vi "Carica sensori canale.vi"(7 "knob":refnum<vi>[](array[refnum]), 8 "error in (no error)":errorcluster, 9 "BANCO":i32, 10 "Array 2":refnum<vi>[](array[refnum]), 11 "Array":refnum<vi>[](array[refnum])) -> (0 "canale--sensore":string[][](array[string]), 1 "sens mand-asp-premist":T2(array[cluster]), 2 "Portate":T2(array[cluster]), 4 "SOMMA":bool)   [LabVIEW 2019]
uses:
  <vilib>/Utility/file.llb/Read Delimited Spreadsheet (string).vi
panel:
  in  "Unità di Misura":T1
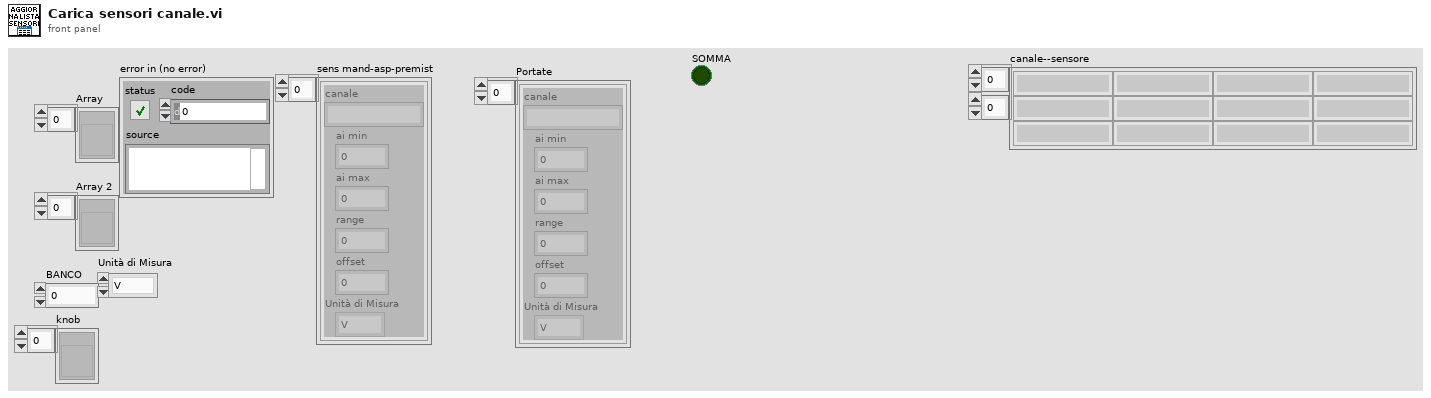
[diagram p1: front panel]
types:
  T1 = typedef "UnitàMisura.ctl" = enum16{"V", "mA", "Bar", "RPM", "m3/s", "m3/min", "m3/h", "l/s", "l/min", "in3/min", "ft3/min", "gpm", "igpm", "igph", "%", "°C", "m", "Nm", "A"}
  T2 = cluster{"canale":string, "ai min":dbl, "ai max":dbl, "range":dbl, "offset":dbl, "Unità di Misura":T1}[]
  T3 = cluster{"canale":string, "ai min":dbl, "ai max":dbl, "range":dbl, "offset":dbl, "Unità di Misura":T1}
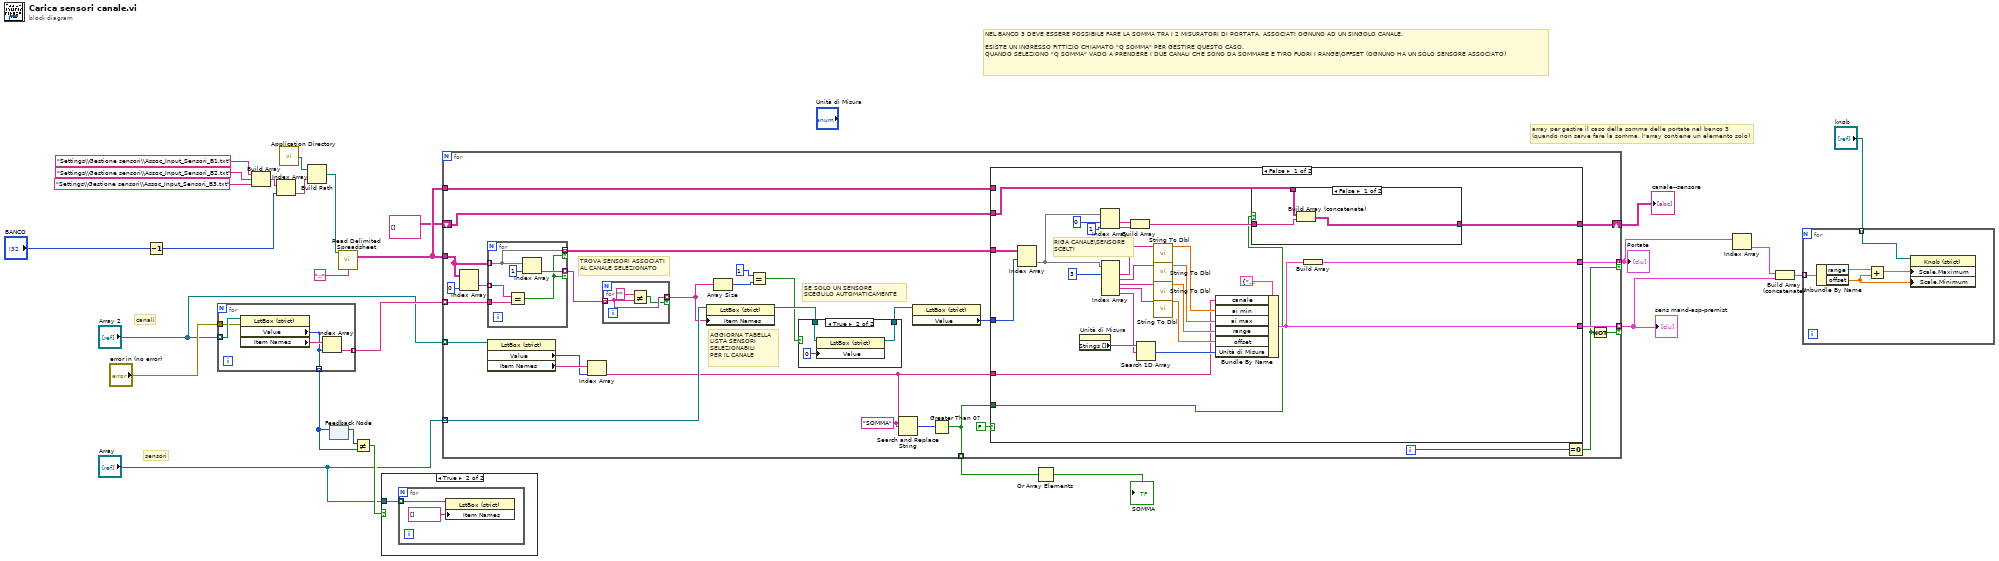
[diagram p0: block diagram]
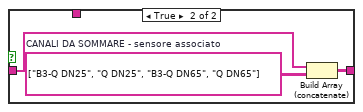
[diagram p3: hidden frame]
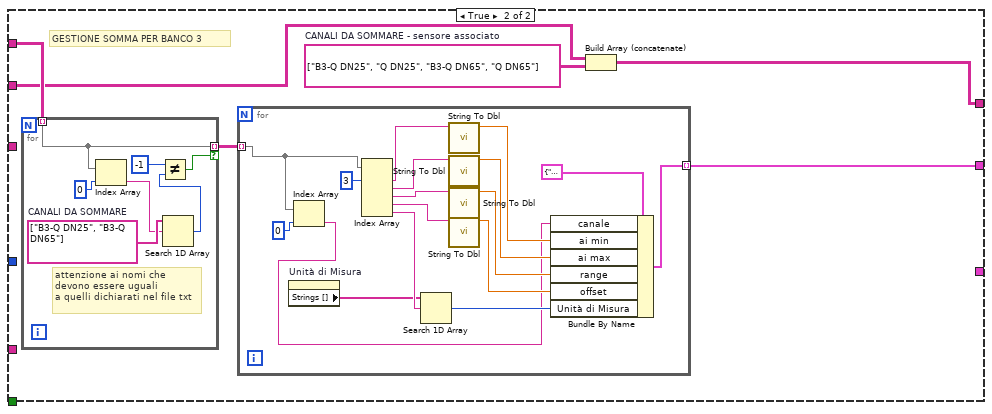
[diagram p4: hidden frame]
diagram:
  # "array per gestire il caso della somma delle portate nel banco 3\n(quando non serve fare la somma, l'array contiene un elemento solo)"
  # "NEL BANCO 3 DEVE ESSERE POSSIBILE FARE LA SOMMA TRA I 2 MISURATORI DI PORTATA, ASSOCIATI OGNUNO AD UN SINGOLO CANALE.\n\nESISTE UN INGRESSO FITTIZIO CHIAMATO \"Q SOMMA\" PER GESTIRE QUESTO CASO.\nQUANDO SELEZIONO \"Q SOMMA\" VADO A PRENDERE I DUE CANALI CHE SONO DA SOMMARE E TIRO FUORI I RANGE\\OFFSET (OGNUNO HA UN SOLO SENSORE ASSOCIATO)"
  # "sensori"
  # "canali"
  n1 = Decrement(x="BANCO") -> (x-1=w13:i32)
  n2 = for {
    tunnel: "Array 2" -> [w32] mode=indexing
    tunnel: [w30] -> w22 mode=indexing
    tunnel: [w29] -> w25 mode=indexing
    tunnel: "error in (no error)" -> [w28]
    n3 = property class="LstBox (strict)"(reference=w32, error in=w28) -> ("Value"=w29:i32, "Item Names"=w31:string[])  [unwired: 2 out]
    n4 = Index Array(array=w31, index=w29) -> (element=w30:string)
  }
  n5 = Build Array("Settings\\Gestione sensori\\Assoc_Input_Sensori_B1.txt" ("name or relative path"), "Settings\\Gestione sensori\\Assoc_Input_Sensori_B2.txt" ("name or relative path"), "Settings\\Gestione sensori\\Assoc_Input_Sensori_B3.txt" ("name or relative path")) -> (w20:string[])
  n6 = Index Array(array=w20, index=w13) -> (element=w16:string)
  n7 = call <vilib>:"Application Directory.vi"() -> ("Application Directory"=w17:path)
  n8 = Build Path(base path=w17, name or relative path=w16) -> (appended path=w15:path)
  n9 = feedback #1() -> (w24:i32[])  [unwired: 1 in]
  n10 = feedback-in #1(w25) -> ()
  n11 = call-poly <vilib>:"Read Delimited Spreadsheet.vi"("file path (dialog if empty)"=w15, "delimiter (\\t)"="::" ("delimiter (\\t)")) -> ("all rows"=w10:string[][])  [unwired: 8 in, 5 out]
  n12 = Not Equal?(x=w24, y=w25) -> (x != y?=w27:bool)
  n13 = case shown="True" w27 {
    tunnel: "Array" -> [_ w33]
    frame False {
    }
    frame True {
      n14 = for {
        tunnel: w33 -> [w35] mode=indexing
        n15 = property class="LstBox (strict)"(reference=w35, "Item Names"=string[] []) -> ()  [unwired: 1 in, 2 out]
      }
    }
  }
  n16 = for {
    tunnel: "Array" -> [w61] mode=indexing
    tunnel: w10 -> [w62]
    tunnel: w22 -> [w65] mode=indexing
    tunnel: [w60] -> w3 mode=indexing if=w41
    tunnel: "Array 2" -> [w50] mode=indexing
    tunnel: [w44] -> w5 mode=concatenating if=w42
    tunnel: w10 -> [w40]
    shift-right: [w39] -> w8
    shift-left: string[][] [] -> [w38]
    tunnel: [w36] -> w7 mode=indexing
    i -> [w43]
    w46 = "SOMMA" ("search string")
    # "SE SOLO UN SENSORE\nSCEGLILO AUTOMATICAMENTE"
    # "AGGIORNA TABELLA\nLISTA SENSORI\nSELEZIONABILI\nPER IL CANALE"
    # "TROVA SENSORI ASSOCIATI\nAL CANALE SELEZIONATO"
    n17 = Index Array(array=w62, index (col)=0 ("index")) -> (element=w63:string[])  [unwired: 1 in]
    n18 = for {
      tunnel: w65 -> [w141]
      tunnel: w63 -> [w140] mode=indexing
      tunnel: w62 -> [w137] mode=indexing
      tunnel: [w138] -> w52 mode=indexing if=w136
      tunnel: [w137] -> w59 mode=indexing if=w136
      n19 = Equal?(x=w140, y=w141) -> (x = y?=w136:bool)
      n20 = Index Array(array=w137, index=1) -> (element=w138:string)
    }
    n21 = property class="LstBox (strict)"(reference=w50) -> ("Value"=w48:i32, "Item Names"=w49:string[])  [unwired: 1 in, 2 out]
    n22 = Index Array(array=w49, index=w48) -> (element=w47:string)
    n23 = for {
      tunnel: w52 -> [w130] mode=indexing
      tunnel: [w130] -> w51 mode=indexing if=w129
      n24 = Not Equal?(x="", y=w130) -> (x != y?=w129:bool)
    }
    n25 = property class="LstBox (strict)"(reference=w61, "Item Names"=w51) -> (reference out=w57:refnum<vi>)  [unwired: 1 in, 1 out]
    n26 = Array Size(array=w51) -> (size(s)=w55:i32)
    n27 = Equal?(x=1, y=w55) -> (x = y?=w53:bool)
    n28 = case shown="True" w53 {
      tunnel: w57 -> [w132 w135]
      tunnel: [w132 w134] -> w56
      frame False {
      }
      frame True {
        n29 = property class="LstBox (strict)"(reference=w135, "Value"=0) -> (reference out=w134:refnum<vi>)  [unwired: 1 in, 1 out]
      }
    }
    n30 = Search and Replace String(input string=w47, search string=w46, replace string=w46) -> (number of replacements=w45:i32)  [unwired: 5 in, 3 out]
    n31 = property class="LstBox (strict)"(reference=w56) -> ("Value"=w58:i32)  [unwired: 1 in, 2 out]
    n32 = Greater Than 0?(x=w45) -> (x > 0?=w36:bool)
    n33 = case shown="False" FALSE {
      tunnel: [w76 _] -> w60
      tunnel: w59 -> [w91 _]
      tunnel: w58 -> [w90 _]
      tunnel: w47 -> [w77 _]
      tunnel: [w75 w99] -> w44
      tunnel: w40 -> [_ w103]
      tunnel: [w67 w101] -> w39
      tunnel: w38 -> [w69 w100]
      tunnel: w36 -> [w66 _]
      frame False {
        # "RIGA CANALE\\SENSORE\nSCELTI"
        n34 = Index Array(array=w91, index (row)=w90) -> (element=w74:string[])  [unwired: 1 in]
        n35 = property on="Unità di Misura" class="Enum (strict)"() -> ("Strings []"=w86:string[])  [unwired: 2 in, 2 out]
        n36 = Index Array(array=w74, index #1=0 ("index"), index #2=1 ("index")) -> (element #1=w70:string, element #2=w71:string)
        n37 = Index Array(array=w74, index #1=3 ("index")) -> (element #1=w88:string, element #2=w83:string, element #3=w81:string, element #4=w79:string, element #5=w85:string)  [unwired: 4 in]
        n38 = Build Array(w70, w71) -> (w68:string[])
        n39 = Search 1D Array(1D array=w86, element=w85) -> (index of element=w84:i32)  [unwired: 1 in]
        n40 = call "String To Dbl.vi"("String"=w88) -> ("Numeric"=w87:dbl)  [unwired: 10 in]
        n41 = call "String To Dbl.vi"("String"=w83) -> ("Numeric"=w82:dbl)  [unwired: 10 in]
        n42 = call "String To Dbl.vi"("String"=w81) -> ("Numeric"=w80:dbl)  [unwired: 10 in]
        n43 = call "String To Dbl.vi"("String"=w79) -> ("Numeric"=w78:dbl)  [unwired: 10 in]
        n44 = Bundle By Name(cluster=T3 {"canale"="", "ai min"=0.0, "ai max"=0.0, "range"=0.0, "offset"=0.0, "Unità di Misura"=enum."V"} ("portata"), "canale"=w77, "ai min"=w87, "ai max"=w82, "range"=w80, "offset"=w78, "Unità di Misura"=w84) -> (w76:T3)
        n45 = case shown="False" w66 {
          tunnel: w69 -> [w95 _]
          tunnel: w68 -> [w94 w97]
          tunnel: [w93 w96] -> w67
          frame False {
            n46 = Build Array (concatenate)(w95, w94) -> (w93:string[][])
          }
          frame True {
            w98 = string[][] [["B3-Q DN25", "Q DN25"], ["B3-Q DN65", "Q DN65"]]  # CANALI DA SOMMARE - sensore associato
            n47 = Build Array (concatenate)(w97, w98) -> (w96:string[][])
          }
        }
        n48 = Build Array(w76) -> (w75:T2)
      }
      frame True {
        w102 = string[][] [["B3-Q DN25", "Q DN25"], ["B3-Q DN65", "Q DN65"]]  # CANALI DA SOMMARE - sensore associato
        # "GESTIONE SOMMA PER BANCO 3"
        n49 = for {
          tunnel: [w105] -> w104 mode=indexing if=w108
          tunnel: w103 -> [w105] mode=indexing
          w110 = string[] ["B3-Q DN25", "B3-Q DN65"]  # CANALI DA SOMMARE
          # "attenzione ai nomi che \ndevono essere uguali\na quelli dichiarati nel file txt"
          n50 = Index Array(array=w105, index=0) -> (element=w109:string)
          n51 = Search 1D Array(1D array=w110, element=w109) -> (index of element=w107:i32)  [unwired: 1 in]
          n52 = Not Equal?(x=-1, y=w107) -> (x != y?=w108:bool)
        }
        n53 = for {
          tunnel: [w116] -> w99 mode=indexing
          tunnel: w104 -> [w114] mode=indexing
          n54 = property on="Unità di Misura" class="Enum (strict)"() -> ("Strings []"=w112:string[])  [unwired: 2 in, 2 out]
          n55 = Index Array(array=w114, index=0) -> (element=w113:string)
          n56 = Index Array(array=w114, index #1=3 ("index")) -> (element #1=w126:string, element #2=w122:string, element #3=w120:string, element #4=w118:string, element #5=w124:string)  [unwired: 4 in]
          n57 = Search 1D Array(1D array=w112, element=w124) -> (index of element=w123:i32)  [unwired: 1 in]
          n58 = call "String To Dbl.vi"("String"=w126) -> ("Numeric"=w125:dbl)  [unwired: 10 in]
          n59 = call "String To Dbl.vi"("String"=w122) -> ("Numeric"=w121:dbl)  [unwired: 10 in]
          n60 = call "String To Dbl.vi"("String"=w120) -> ("Numeric"=w119:dbl)  [unwired: 10 in]
          n61 = call "String To Dbl.vi"("String"=w118) -> ("Numeric"=w117:dbl)  [unwired: 10 in]
          n62 = Bundle By Name(cluster=T3 {"canale"="", "ai min"=0.0, "ai max"=0.0, "range"=0.0, "offset"=0.0, "Unità di Misura"=enum."V"} ("portata"), "canale"=w113, "ai min"=w125, "ai max"=w121, "range"=w119, "offset"=w117, "Unità di Misura"=w123) -> (w116:T3)
        }
        n63 = Build Array (concatenate)(w100, w102) -> (w101:string[][])
      }
    }
    n64 = Equal To 0?(x=w43) -> (x = 0?=w42:bool)
    n65 = Not(x=w42) -> (.not. x?=w41:bool)
  }
  "sens mand-asp-premist" <- w3
  "Portate" <- w5
  "canale--sensore" <- w8
  n66 = Or Array Elements(Boolean array=w7) -> (logical OR=→"SOMMA":bool)
  n67 = Index Array(array=w5) -> (element=w4:T3)  [unwired: 1 in]
  n68 = Build Array (concatenate)(w4, w3) -> (w2:T2)
  n69 = for {
    tunnel: w2 -> [w146] mode=indexing
    tunnel: "knob" -> [w145] mode=indexing
    n70 = Unbundle By Name(w146) -> ("range"=w144:dbl, "offset"=w142:dbl)
    n71 = Add(x=w144, y=w142) -> (x+y=w143:dbl)
    n72 = property class="Knob (strict)"(reference=w145, "Scale.Maximum"=w143, "Scale.Minimum"=w142) -> ()  [unwired: 1 in, 2 out]
  }
